vi "TSLoadFile.vi"(0 "Path":path) -> (4 "Trap":dbl[][](array[numeric]) format="%_3g", 6 "TPos":dbl[][](array[numeric]) format="%.2f", 8 "Fluor":u16[][](array[numeric]), 12 "Hdr":dbl[](array[numeric]), 13 "TPos Hdr":dbl[](array[numeric]), 14 "Fl Hdr":dbl[](array[numeric]), 15 "Fs":dbl)   [LabVIEW 2014]
panel:
  out "Cmt":string
  # "On Flzr it's:\n'AY' 'AX' 'AS' 'BY' 'BX' 'BS' 'AFbX' 'AFbS' 'BFbX' 'BFbS' 'CY' 'CX' 'SCY' 'SCX'"
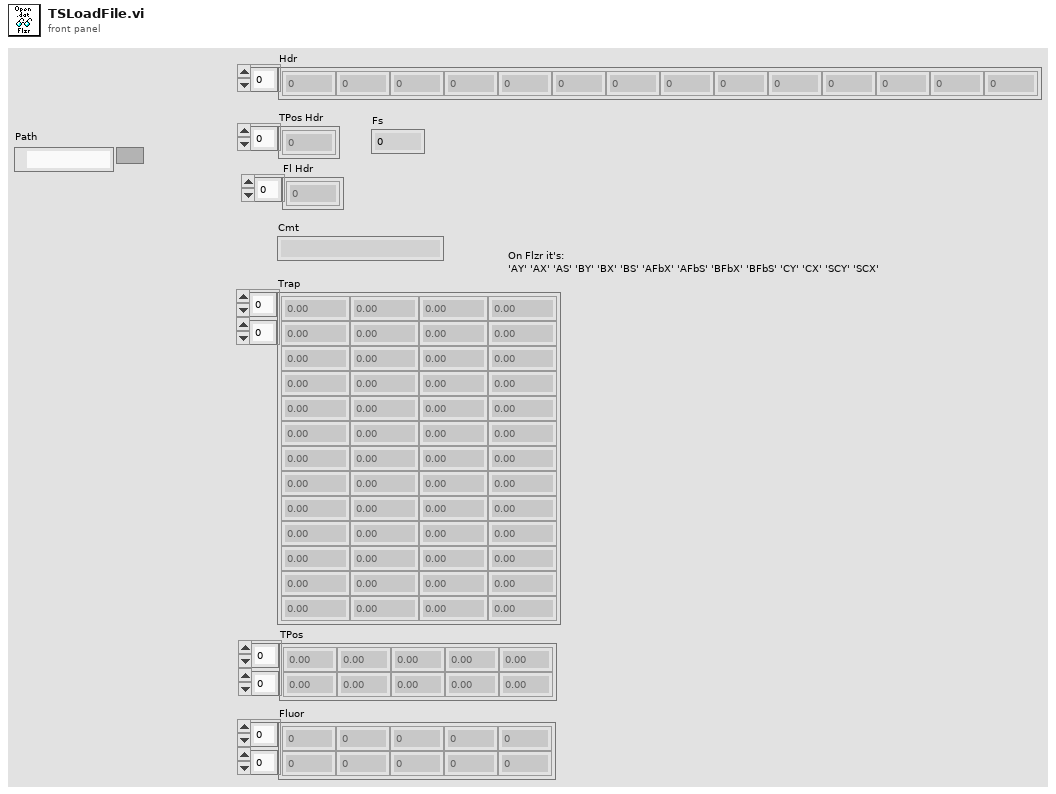
[diagram p1: front panel]
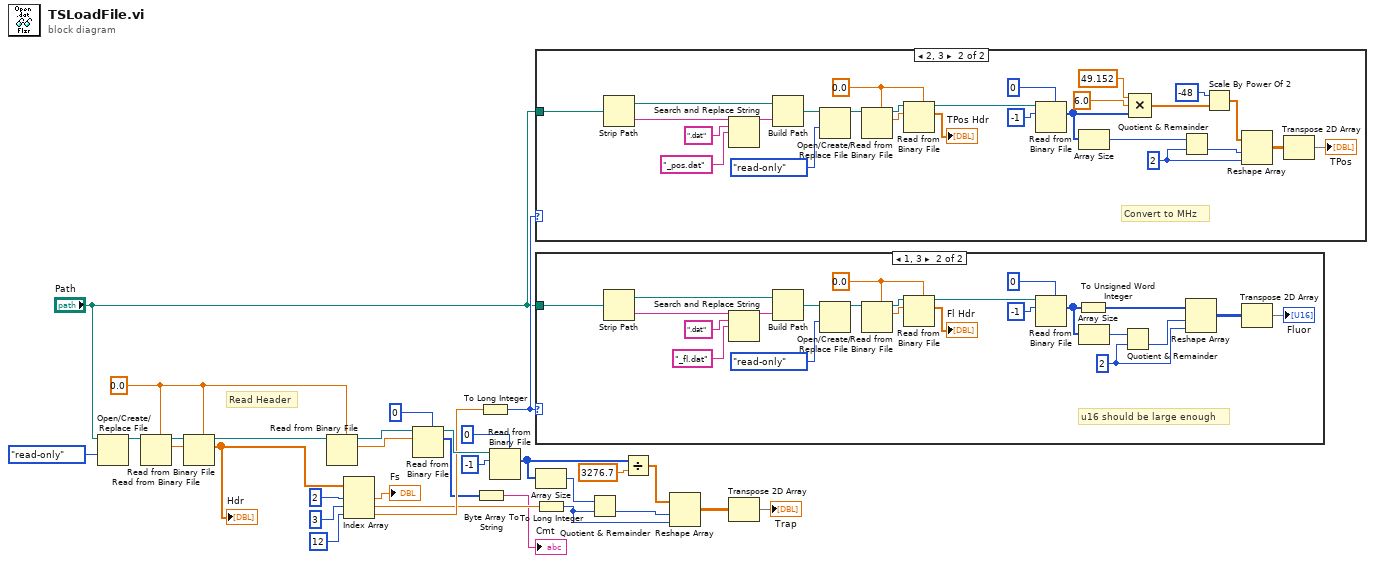
[diagram p0: block diagram]
diagram:
  w9 = 0.0
  # "Read Header"
  n1 = Open/Create/Replace File(file path (use dialog)="Path", access (0:read/write)=enum16{"read/write", "read-only", "write-only"}."read-only") -> (refnum out=w30:refnum<file>)  [unwired: 4 in, 2 out]
  n2 = Read from Binary File(5:w9, 11:w30) -> (2:w29:dbl, 3:w28:refnum<file>)  [unwired: 4 in, 2 out]
  n3 = Read from Binary File(5:w9, 10:w29, 11:w28) -> (2:w23:dbl[], 3:w25:refnum<file>)  [unwired: 3 in, 2 out]
  "Hdr" <- w23
  n4 = Read from Binary File(5:w9, 11:w25) -> (2:w26:dbl, 3:w27:refnum<file>)  [unwired: 4 in, 2 out]
  n5 = Index Array(array=w23, index #1=2 ("index"), index #2=3 ("index"), index #3=12 ("index")) -> (element #1=→"Fs":dbl, element #2=w12:dbl, element #3=w16:dbl)
  n6 = Read from Binary File(5:u8 0, 10:w26, 11:w27) -> (2:w4:u8[], 3:w24:refnum<file>)  [unwired: 3 in, 2 out]
  n7 = Byte Array To String(unsigned byte array=w4) -> (string=→"Cmt":string)
  n8 = To Long Integer(number=w16) -> (32bit integer=w15:i32)
  n9 = Read from Binary File(5:i16 0, 10:-1 ("count (1)"), 11:w24) -> (2:w6:i16[])  [unwired: 3 in, 3 out]
  n10 = case shown="2, 3" w15 {
    tunnel: "Path" -> [_ w58]
    frame 0, Default {
    }
    frame 2, 3 {
      w41 = 2 ("dimension size")
      w52 = 0.0
      # "Convert to MHz"
      n11 = Strip Path(path=w58) -> (stripped path=w57:path, name=w56:string)
      n12 = Search and Replace String(input string=w56, search string=".dat", replace string="_pos.dat" ("replace string (\"\")")) -> (result string=w53:string)  [unwired: 5 in, 3 out]
      n13 = Build Path(base path=w57, name or relative path=w53) -> (appended path=w47:path)
      n14 = Open/Create/Replace File(file path (use dialog)=w47, access (0:read/write)=enum16{"read/write", "read-only", "write-only"}."read-only") -> (refnum out=w49:refnum<file>)  [unwired: 4 in, 2 out]
      n15 = Read from Binary File(5:w52, 11:w49) -> (2:w50:dbl, 3:w51:refnum<file>)  [unwired: 4 in, 2 out]
      n16 = Read from Binary File(5:w52, 10:w50, 11:w51) -> (2:→"TPos Hdr":dbl[], 3:w44:refnum<file>)  [unwired: 3 in, 2 out]
      n17 = Read from Binary File(5:u64 0, 10:-1 ("count (1)"), 11:w44) -> (2:w34:u64[])  [unwired: 3 in, 3 out]
      n18 = Array Size(array=w34) -> (size(s)=w39:i32)
      n19 = Compound Arithmetic op=MULTIPLY(49.152, 6.0, w34) -> (w36:dbl[])
      n20 = Quotient & Remainder(x=w39, y=w41) -> (floor(x/y)=w40:i32)  [unwired: 1 out]
      n21 = Scale By Power Of 2(n=i16 -48, x=w36) -> (x*2^n=w33:dbl[])
      n22 = Reshape Array(w33, w40, w41) -> (w43:dbl[][])
      n23 = Transpose 2D Array(2D array=w43) -> (transposed array=→"TPos":dbl[][])
    }
  }
  n24 = case shown="1, 3" w15 {
    tunnel: "Path" -> [_ w81]
    frame 0, Default {
    }
    frame 1, 3 {
      w63 = 2 ("dimension size")
      w75 = 0.0
      # "u16 should be large enough"
      n25 = Strip Path(path=w81) -> (stripped path=w80:path, name=w79:string)
      n26 = Search and Replace String(input string=w79, search string=".dat", replace string="_fl.dat" ("replace string (\"\")")) -> (result string=w76:string)  [unwired: 5 in, 3 out]
      n27 = Build Path(base path=w80, name or relative path=w76) -> (appended path=w70:path)
      n28 = Open/Create/Replace File(file path (use dialog)=w70, access (0:read/write)=enum16{"read/write", "read-only", "write-only"}."read-only") -> (refnum out=w72:refnum<file>)  [unwired: 4 in, 2 out]
      n29 = Read from Binary File(5:w75, 11:w72) -> (2:w73:dbl, 3:w74:refnum<file>)  [unwired: 4 in, 2 out]
      n30 = Read from Binary File(5:w75, 10:w73, 11:w74) -> (2:→"Fl Hdr":dbl[], 3:w67:refnum<file>)  [unwired: 3 in, 2 out]
      n31 = Read from Binary File(5:u64 0, 10:-1 ("count (1)"), 11:w67) -> (2:w64:u64[])  [unwired: 3 in, 3 out]
      n32 = To Unsigned Word Integer(number=w64) -> (unsigned 16bit integer=w60:u16[])
      n33 = Array Size(array=w64) -> (size(s)=w62:i32)
      n34 = Quotient & Remainder(x=w62, y=w63) -> (floor(x/y)=w61:i32)  [unwired: 1 out]
      n35 = Reshape Array(w60, w61, w63) -> (w66:u16[][])
      n36 = Transpose 2D Array(2D array=w66) -> (transposed array=→"Fluor":u16[][])
    }
  }
  n37 = Array Size(array=w6) -> (size(s)=w13:i32)
  n38 = To Long Integer(number=w12) -> (32bit integer=w10:i32)
  n39 = Quotient & Remainder(x=w13, y=w10) -> (floor(x/y)=w11:i32)  [unwired: 1 out]
  n40 = Divide(x=w6, y=3276.7) -> (x/y=w5:dbl[])
  n41 = Reshape Array(w5, w11, w10) -> (w18:dbl[][])
  n42 = Transpose 2D Array(2D array=w18) -> (transposed array=→"Trap":dbl[][])
